vi "寻找拐点.vi"(8 "POINT":dbl, 9 "偏移量":i32, 10 "数组":dbl[](array[numeric]), 11 "二阶导数":dbl[](array[numeric])) -> (0 "拐点索引":i32, 1 "拐点值":dbl, 3 "起点":i32)   [LabVIEW 2011]
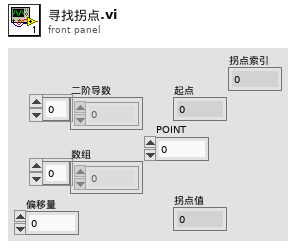
[diagram p1: front panel]
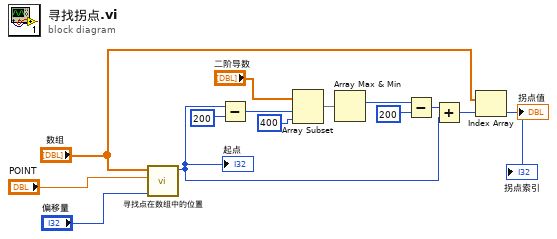
[diagram p0: block diagram]
diagram:
  n1 = call "寻找点在数组中的位置.vi"("偏移量"="偏移量", "x"="POINT", "数组"="数组") -> ("起点"=w12:i32)  [unwired: 8 in]
  "起点" <- w12
  n2 = Subtract(x=w12, y=200) -> (x-y=w4:i32)
  n3 = Array Subset(array="二阶导数", index=w4, length=400 ("长度")) -> (w6:dbl[])
  n4 = Array Max & Min(array=w6) -> (max index (indices)=w9:i32)  [unwired: 3 out]
  n5 = Subtract(x=w9, y=200) -> (x-y=w11:i32)
  n6 = Add(x=w11, y=w12) -> (x+y=w14:i32)
  "拐点索引" <- w14
  n7 = Index Array(array="数组", index=w14) -> (element=→"拐点值":dbl)
